vi "resetTempFolder.vi"   [LabVIEW 2012]
uses:
  GlobalBaslerCamera.vi
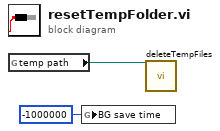
[diagram p0: block diagram]
diagram:
  n1 = global read "GlobalBaslerCamera.vi" "temp path"() -> (w2:path)
  n2 = global write "GlobalBaslerCamera.vi" "BG save time"(i64 -1000000 ("BG save time")) -> ()
  n3 = call "deleteTempFiles.vi"("path"=w2) -> ()  [unwired: 8 in, 1 out]
